vi "Init.vi"(8 "error in (no error)":errorcluster, 10 "Channel":i16, 11 "TrialBasedExperiment in":refnum<class "MouseDotMapping.lvclass">) -> (0 "error out":errorcluster, 3 "TrialBasedExperiment out":refnum<class "MouseDotMapping.lvclass">)   [LabVIEW 2014, in "MouseDotMapping.lvclass"]
uses:
  MouseDotMapping.lvclass
  Trial Based Experiment Statechart/PassiveExperiment/PassiveExperiment.lvclass
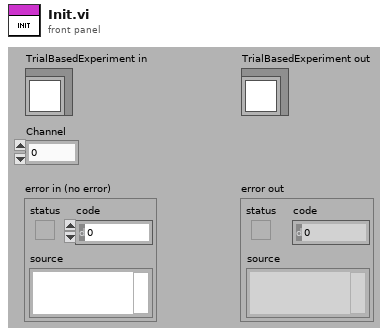
[diagram p1: front panel]
types:
  T1 = cluster{"Intertrial":dbl, "AcquireFixation":dbl, "HoldFixation":dbl, "DelayPeriod":dbl, "ResponsePeriod":dbl}
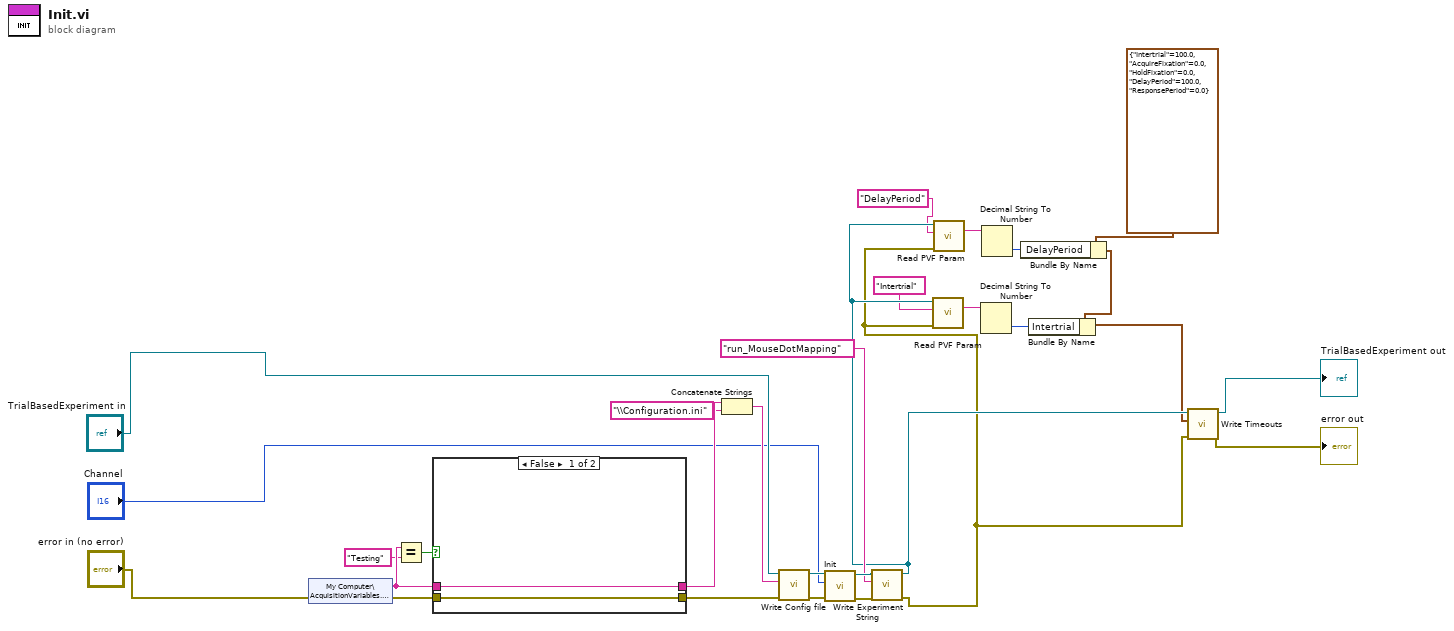
[diagram p0: block diagram]
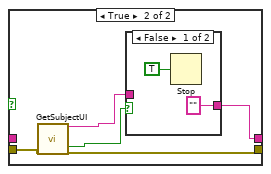
[diagram p2: hidden frame]
diagram:
  n1 = shared-variable "My Computer\\AcquisitionVariables.lvlib\\Subject"(error in="error in (no error)") -> (w21:string, error out=w22:errorcluster)
  n2 = Equal?(x=w21, y="Testing") -> (x = y?=w19:bool)
  n3 = case shown="False" w19 {
    tunnel: [w31 w36] -> w25
    tunnel: w21 -> [w31 _]
    tunnel: w22 -> [w30 w32]
    tunnel: [w30 w33] -> w23
    frame False {
    }
    frame True {
      n4 = call "GetSubjectUI.vi"("error in (no error)"=w32) -> ("subjectSelected"=w35:string, "OK"=w34:bool, "error out"=w33:errorcluster)  [unwired: 16 in]
      n5 = case shown="False" w34 {
        tunnel: w35 -> [_ w39]
        tunnel: ["" ("subjectSelected") w39] -> w36
        frame False {
          n6 = Stop(stop? (T)=TRUE) -> ()
        }
        frame True {
        }
      }
    }
  }
  n7 = Concatenate Strings(w25, "\\Configuration.ini") -> (w17:string)
  n8 = call-dynamic "Write Config file.vi"("error in (no error)"=w23, "Config file"=w17, "TrialBasedExperiment in"="TrialBasedExperiment in") -> ("error out"=w27:errorcluster, "TrialBasedExperiment out"=w26:refnum<class "MouseDotMapping.lvclass">)  [unwired: 7 in]
  n9 = call-parent "Init.vi"("error in (no error)"=w27, "Channel"="Channel", "TrialBasedExperiment in"=w26) -> ("error out"=w29:errorcluster, "TrialBasedExperiment out"=w28:refnum<class "MouseDotMapping.lvclass">)  [unwired: 7 in]
  n10 = call-dynamic "Write Experiment String.vi"("error in (no error)"=w29, "Experiment String"="run_MouseDotMapping" ("string"), "TrialBasedExperiment in"=w28) -> ("error out"=w4:errorcluster, "TrialBasedExperiment out"=w5:refnum<class "MouseDotMapping.lvclass">)  [unwired: 7 in]
  n11 = call-dynamic "Read PVF Param.vi"("error in (no error)"=w4, "Param Name"="Intertrial", "MatlabExperiment in"=w5) -> ("Param Value"=w10:string)  [unwired: 6 in, 2 out]
  n12 = call-dynamic "Read PVF Param.vi"("error in (no error)"=w4, "Param Name"="DelayPeriod", "MatlabExperiment in"=w5) -> ("Param Value"=w8:string)  [unwired: 6 in, 2 out]
  n13 = Decimal String To Number(string=w10) -> (number=w11:i32)  [unwired: 2 in, 1 out]
  n14 = Decimal String To Number(string=w8) -> (number=w9:i32)  [unwired: 2 in, 1 out]
  n15 = Bundle By Name(cluster=T1 {"Intertrial"=100.0, "AcquireFixation"=0.0, "HoldFixation"=0.0, "DelayPeriod"=100.0, "ResponsePeriod"=0.0} ("Timeouts"), "DelayPeriod"=w9) -> (w12:T1)
  n16 = Bundle By Name(cluster=w12, "Intertrial"=w11) -> (w3:T1)
  n17 = call-dynamic "Write Timeouts.vi"("error in (no error)"=w4, "Timeouts"=w3, "TrialBasedExperiment in"=w5) -> ("error out"=→"error out":errorcluster, "TrialBasedExperiment out"=→"TrialBasedExperiment out":refnum<class "MouseDotMapping.lvclass">)  [unwired: 7 in]
